vi "TIFF-BlockAvgStdContrast.vi"(1 "Theshold":dbl=200.0, 4 "Output file":u16(ring)=1 items=["Big-Endian"=0, "Native"=1, "Little-Endian"=2, "BigTiff-Big-Endian"=256, "Bigtiff,Native"=257, "Biftiff,Littleendian"=258], 5 "offset":dbl=3200.0, 7 "Enum":enum16{"AVG", "STD", "Contrast1000"}(ring), 8 "Stop at offset:":u64=4294967295, 9 "Blocksize":i16=8, 10 "inputfile":path) -> (3 "File out":path)   [LabVIEW 2011]
uses:
  tiff/TiffModules/AddTiffPage_U16_text_res.vi
panel:
  out "Block":i32
  out "AfterDIRoffset":u32 format="%09d"
  out "Input-page":i32
  out "Out":u16[][](graph)
  out "In":u16[][](graph)
  # "select raw tiff file\nselect blocksize, method\nrun\nnew name first with _<type>.tif\nstops at max tiff-offset 2^32\nContrast need offset (%) and threshold (darunter 0)"
  # "max-min"
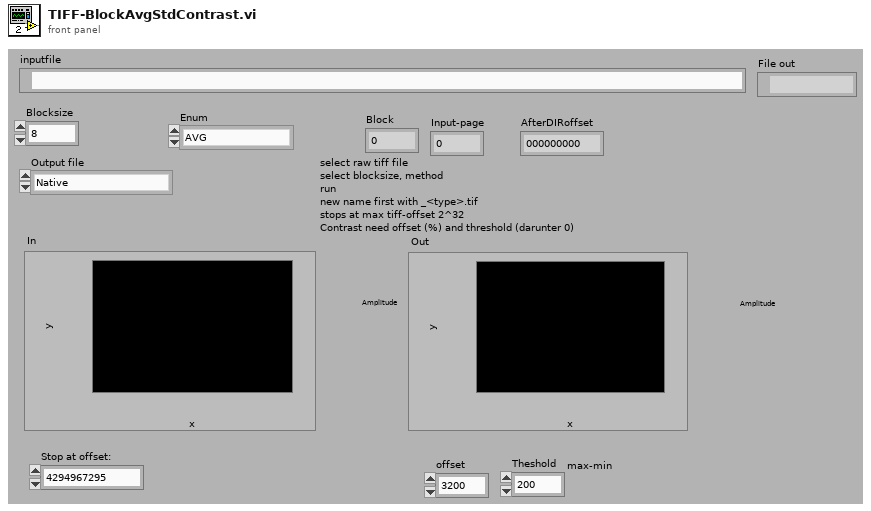
[diagram p1: front panel]
types:
  T1 = cluster{"Tiff refnum":refnum<file>, "BigTiff,Endian":u16}
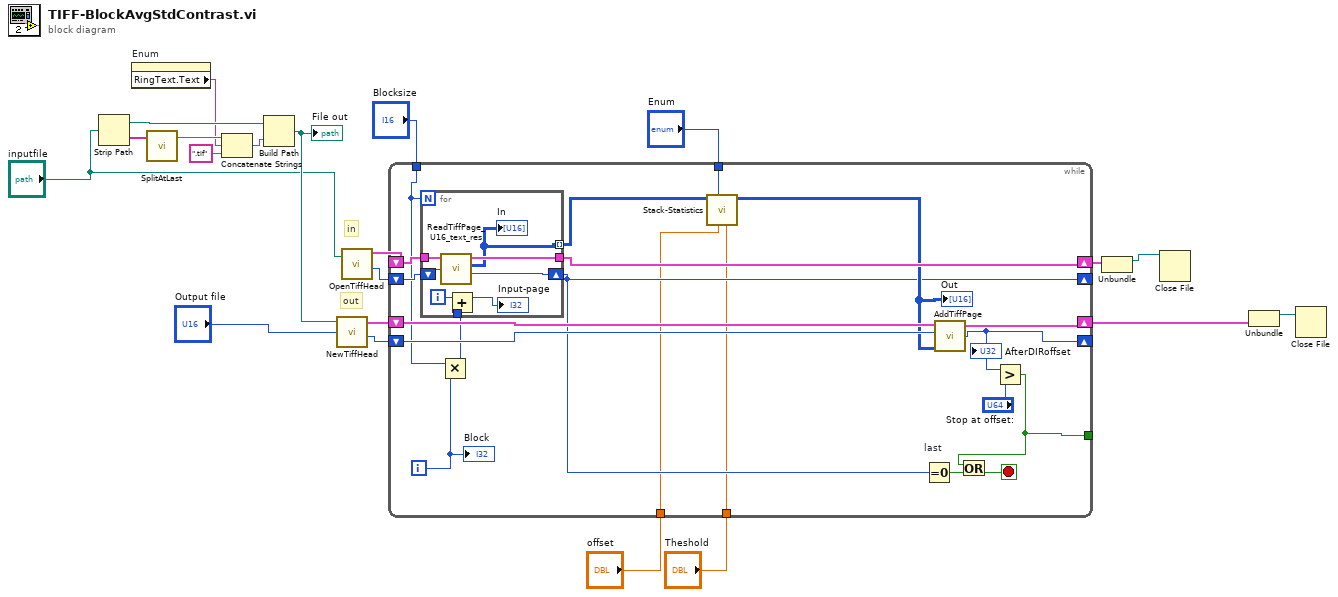
[diagram p0: block diagram]
diagram:
  # "out"
  # "in"
  n1 = Strip Path(path="inputfile") -> (stripped path=w13:path, name=w14:string)
  n2 = property on="Enum" class="Enum (strict)"() -> ("RingText.Text"=w11:string)  [unwired: 2 in, 2 out]
  n3 = call "SplitAtLast.vi"("In-String"=w14) -> ("Front (default)"=w15:string)  [unwired: 1 in, 1 out]
  n4 = Concatenate Strings(w15, w11, ".tif" ("string")) -> (w21:string)
  n5 = Build Path(base path=w13, name or relative path=w21) -> (appended path=w20:path)
  "File out" <- w20
  n6 = call "NewTiffHead.vi"("file path"=w20, "BigTiff,Endian"="Output file") -> ("TIFF file"=w19:T1, "Place for first IFD (8,eof-position)"=w18:u64)  [unwired: 2 in, 1 out]
  n7 = call "OpenTiffHead.vi"("file path"="inputfile") -> ("TIFF file"=w9:T1, "first Diroffset"=w8:u64)  [unwired: 2 in, 1 out]
  n8 = while {
    shift-right: [w35] -> w7
    shift-left: w9 -> [w37]
    shift-right: [w40] -> w17
    shift-left: w19 -> [w41]
    shift-right: [w27] -> _
    shift-left: w8 -> [w36]
    shift-right: [w31] -> _
    shift-left: w18 -> [w39]
    tunnel: [w32] -> _
    tunnel: "Enum" -> [w29]
    tunnel: "Blocksize" -> [w23]
    tunnel: "offset" -> [w26]
    tunnel: "Theshold" -> [w25]
    i -> [w22]
    stop <- w33 stop-if-true
    n9 = Multiply(x=w23, y=w22) -> (x*y=w24:i32)
    n10 = for {
      N: w23 -> [_]
      tunnel: w37 -> [w49]
      tunnel: [w47] -> w35
      tunnel: [w46] -> w30 mode=indexing
      tunnel: w24 -> [w43]
      shift-right: [w42] -> w27
      shift-left: w36 -> [w48]
      i -> [w45]
      n11 = call "ReadTiffPage_U16_text_res.vi"("TIFF file"=w49, "IFDoffset"=w48) -> ("TIFF file out"=w47:T1, "16-bit pixmap"=w46:u16[][], "Next offset"=w42:i64)  [unwired: 3 in, 3 out]
      "In" <- w46
      n12 = Add(x=w45, y=w43) -> (x+y=→"Input-page":i32)
    }
    n13 = call "Stack-Statistics.vi"("Theshold"=w25, "offset"=w26, "Enum"=w29, "16-bit pixmap"=w30) -> ("Out"=w28:u16[][])  [unwired: 7 in]
    "Out" <- w28
    n14 = Equal To 0? "last"(x=w27) -> (x = 0?=w38:bool)
    n15 = call-poly "AddTiffPage.vi"("TIFF file"=w41, "After last DIROffset"=w39, "16-bit pixmap x, y"=w28) -> ("TIFF file"=w40:T1, "AfterDIRoffset"=w31:u64)  [unwired: 2 in, 1 out]
    "AfterDIRoffset" <- w31
    n16 = Greater?(x=w31, y="Stop at offset:") -> (0:w32:bool)
    n17 = Or(x=w32, y=w38) -> (x .or. y?=w33:bool)
    "Block" <- w22
  }
  n18 = Unbundle(w7) -> ("Tiff refnum"=w6:refnum<file>)  [unwired: 1 out]
  n19 = Close File(refnum=w6) -> ()  [unwired: 1 in, 2 out]
  n20 = Unbundle(w17) -> ("Tiff refnum"=w16:refnum<file>)  [unwired: 1 out]
  n21 = Close File(refnum=w16) -> ()  [unwired: 1 in, 2 out]
